vi "Call Emergency.vi"(8 "error in (no error)":errorcluster, 10 "Emergency":bool, 11 "Elevator Controller Actor in":refnum<class "Elevator Controller Actor.lvclass">) -> (0 "error out":errorcluster, 3 "Elevator Controller Actor out":refnum<class "Elevator Controller Actor.lvclass">)   [LabVIEW 2019, in "Elevator Controller Actor.lvlib" / "Elevator Controller Actor.lvclass"]
uses:
  Elevator Controller Actor.lvclass
  Sim Display Console Actor/Sim Display Console Actor Messages/Write Elevator Location Msg/Write Elevator Location Msg.lvclass
  Sim Display Console Actor/Sim Display Console Actor Messages/Write Door Open Msg/Write Door Open Msg.lvclass
  Elevator Controller Actor Messages/Set State Msg/Set State Msg.lvclass
  State -Enum.ctl
  <vilib>/ActorFramework/Actor/Actor.lvclass
  C:/Program Files (x86)/National Instruments/LabVIEW 2019/vi.lib/ActorFramework/Actor/Actor.lvclass
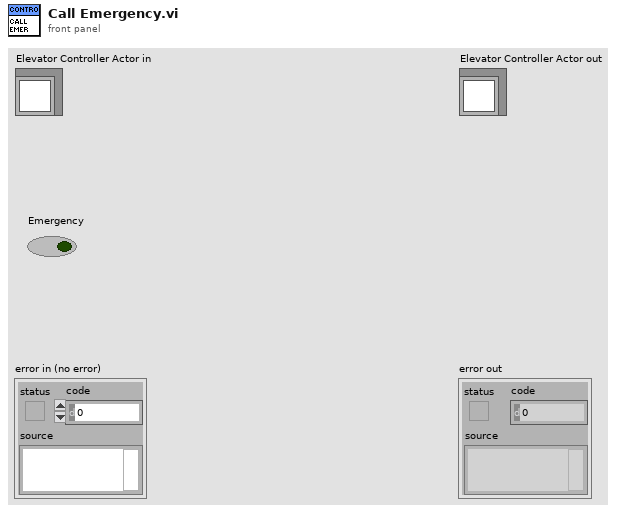
[diagram p1: front panel]
types:
  T1 = typedef "Elevator Controller Actor.lvlib/Elevator Controller Actor.lvclass/State -Enum.ctl" = enum16{"Initial", "Wait for First Request", "Start and Move", "Anaysis", "Continue Travel", "Stop at Floor", "Open and Close Door Sequence", "No Request Remaining", "Emergency Call", "Terminate Process"}
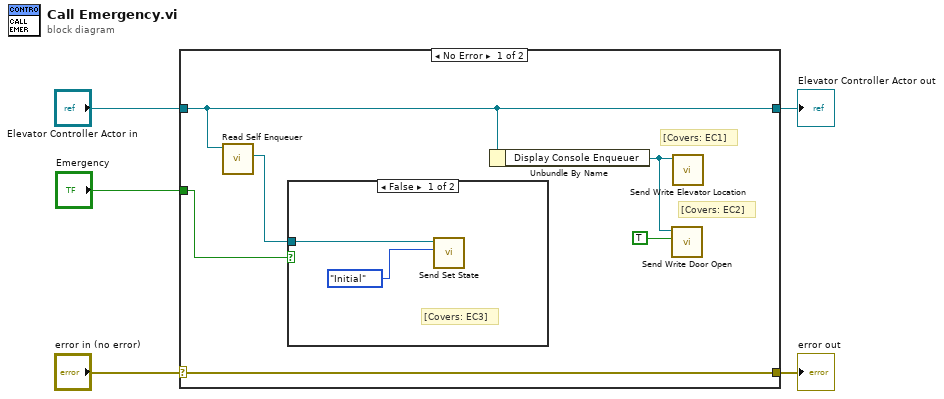
[diagram p0: block diagram]
diagram:
  n1 = case shown="No Error" "error in (no error)" {
    selector: "error in (no error)" -> [w11 w15]
    tunnel: [w11 w15] -> w4
    tunnel: [w7 w14] -> w2
    tunnel: "Elevator Controller Actor in" -> [w7 w14]
    tunnel: "Emergency" -> [w8 _]
    frame No Error {
      # "[Covers: EC2]"
      # "[Covers: EC1]"
      n2 = call <vilib>:"Read Self Enqueuer.vi"("Actor"=w7) -> ("Self Enqueuer"=w6:refnum<class "Message Enqueuer.lvclass">)  [unwired: 10 in]
      n3 = case shown="False" w8 {
        tunnel: w6 -> [w12 _]
        frame False {
          # "[Covers: EC3]"
          n4 = call "Send Set State.vi"("States"=State_-Enum."Initial", "Message Enqueuer"=w12) -> ()  [unwired: 8 in, 2 out]
        }
        frame True {
        }
      }
      n5 = Unbundle By Name(w7) -> ("Display Console Enqueuer"=w10:refnum<class "Message Enqueuer.lvclass">)
      n6 = call "Send Write Door Open.vi"("Door Open"=TRUE, "Message Enqueuer"=w10) -> ()  [unwired: 8 in, 2 out]
      n7 = call "Send Write Elevator Location.vi"("Message Enqueuer"=w10) -> ()  [unwired: 9 in, 2 out]
    }
    frame Error {
    }
  }
  "error out" <- w4
  "Elevator Controller Actor out" <- w2
